vi "Configure Channel.vi"(8 "error in (no error)":errorcluster, 9 "Config Channel":T1={"Channel (0: Channel 1)"=0, "Vertical Coupling (1: DC)"=1, "Probe Attenuation (10: 10X)"=10, "Vertical Range (10.0 V/div)"=10.0, "Vertical Offset (0.0 divs)"=0.0, "Bandwidth (0: MAX Bandwidth)"=0, "Enable Channel (True)"=TRUE} {"Bandwidth (0: MAX Bandwidth)" items=["MAX Bandwidth", "Unlimited"]; "Probe Attenuation (10: 10X)" items=["1"=1, "10"=10, "20"=20, "50"=50, "100"=100, "500"=500, "1000"=1000]; "Vertical Coupling (1: DC)" items=["AC", "DC", "Ground"]; "Channel (0: Channel 1)" items=["Channel 1", "Channel 2", "Channel 3", "Channel 4", "Math", "Reference A", "Reference B", "Reference C", "Reference D"]}, 11 "EDU-X-1002A in":refnum<class "EDU-X-1002A.lvclass">) -> (0 "error out":errorcluster, 3 "EDU-X-1002A out":refnum<class "EDU-X-1002A.lvclass">)   [LabVIEW 2020, in "Controlador.lvlib" / "EDU-X-1002A.lvclass"]
uses:
  EDU-X-1002A.lvclass
  C:/Users/scrap/Fork/Modulo_Cloneable_DQMH/Libraries/Controlador/Class/Osciloscope/Osciloscope.lvclass
  Osciloscope/Osciloscope.lvclass/Osciloscope.ctl
  Osciloscope/Read COM.vi
  <instrlib>/Agilent 2000 3000 X-Series/Agilent 2000 3000 X-Series.lvlib
  Osciloscope/Osciloscope.lvclass
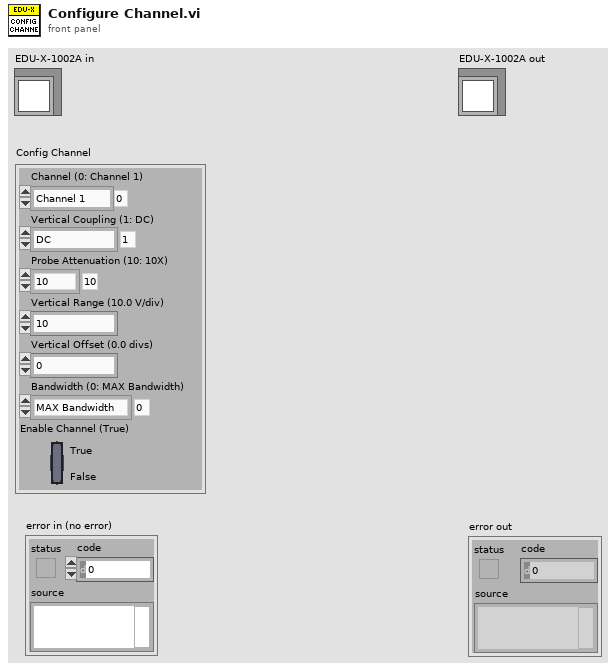
[diagram p1: front panel]
types:
  T1 = cluster{"Channel (0: Channel 1)":i32, "Vertical Coupling (1: DC)":i32, "Probe Attenuation (10: 10X)":i32, "Vertical Range (10.0 V/div)":dbl, "Vertical Offset (0.0 divs)":dbl, "Bandwidth (0: MAX Bandwidth)":i32, "Enable Channel (True)":bool}
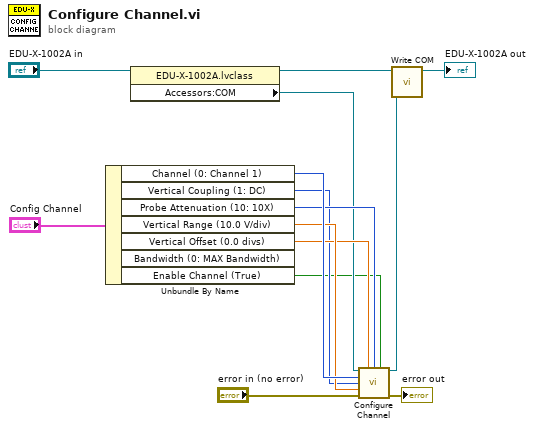
[diagram p0: block diagram]
diagram:
  n1 = Unbundle By Name("Config Channel") -> ("Channel (0: Channel 1)"=w11:i32, "Vertical Coupling (1: DC)"=w7:i32, "Probe Attenuation (10: 10X)"=w10:i32, "Vertical Range (10.0 V/div)"=w9:dbl, "Vertical Offset (0.0 divs)"=w8:dbl, "Enable Channel (True)"=w1:bool)  [unwired: 1 out]
  n2 = property class="EDU-X-1002A.lvclass"(reference="EDU-X-1002A in") -> (reference out=w6:refnum<class "EDU-X-1002A.lvclass">, "Accessors:COM"=w5:refnum<visa-resource-name>)  [unwired: 1 in, 1 out]
  n3 = call <instrlib>:"Configure Channel.vi"("VISA resource name"=w5, "Enable Channel (T: Enable)"=w1, "Channel Name (0: Channel 1)"=w11, "Coupling (1: DC)"=w7, "Vertical Range (40.0 V)"=w9, "error in (no error)"="error in (no error)", "Vertical Offset (0.0)"=w8, "Probe Attenuation (1.0)"=w10) -> ("VISA resource name out"=w4:refnum<visa-resource-name>, "error out"=→"error out":errorcluster)  [unwired: 6 in]
  n4 = call "Write COM.vi"("COM"=w4, "Osciloscope in"=w6) -> ("Osciloscope out"=→"EDU-X-1002A out":refnum<class "EDU-X-1002A.lvclass">)  [unwired: 8 in, 1 out]
